vi "Get Attachments.vi"(6 "Authorization":T2[](array[typedef]), 8 "error in (no error)":errorcluster, 10 "Task GID":string) -> (0 "error out":errorcluster, 1 "data":T1(array[cluster]))   [LabVIEW 2016]
uses:
  <vilib>/addons/_JKI.lib/REST Client/classes/REST Client/HTTP Header.ctl
  <vilib>/addons/_JKI.lib/REST Client/classes/REST Client/REST Client.lvclass
  <vilib>/addons/_JKI.lib/Serialization/JSON/JKI JSON Serialization.lvlib
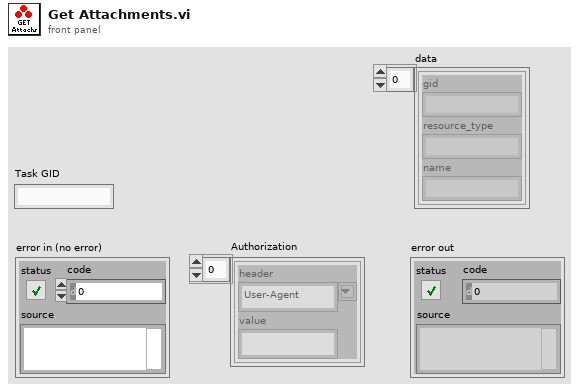
[diagram p1: front panel]
types:
  T1 = cluster{"gid":string, "resource_type":string, "name":string}[]
  T2 = typedef "REST Client.lvlib/REST Client.lvclass/HTTP Header.ctl" = cluster{"header":string, "value":string}
  T3 = cluster{"data":cluster{"gid":string, "resource_type":string, "name":string}[]}
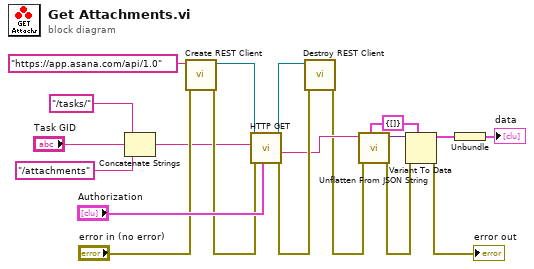
[diagram p0: block diagram]
diagram:
  w3 = T3 {"data"=[]}
  n1 = Concatenate Strings("/tasks/", "Task GID", "/attachments") -> (w14:string)
  n2 = call <vilib>:"Create REST Client.vi"("error in (no error)"="error in (no error)", "Base URL"="https://app.asana.com/api/1.0") -> ("error out"=w15:errorcluster, "REST Client out"=w17:refnum<class "REST Client.lvclass">)  [unwired: 8 in]
  n3 = call-dynamic "HTTP GET.vi"("request specific headers"="Authorization", "error in (no error)"=w15, "Path"=w14, "REST Client in"=w17) -> ("error out"=w10:errorcluster, "Response body"=w8:string, "REST Client out"=w9:refnum<class "REST Client.lvclass">)  [unwired: 2 in, 3 out]
  n4 = call-dynamic "Destroy REST Client.vi"("error in (no error)"=w10, "REST Client in"=w9) -> ("error out"=w7:errorcluster)  [unwired: 9 in]
  n5 = call <vilib>:"Unflatten From JSON String.vi"("Type and Defaults"=w3, "error in (no error)"=w7, "JSON String"=w8) -> ("error out"=w6:errorcluster, "Variant"=w4:variant)  [unwired: 7 in]
  n6 = Variant To Data(error in=w6, type=w3, Variant=w4) -> (data=w2:T3, error out=→"error out":errorcluster)
  n7 = Unbundle(w2) -> ("data"=→"data":T1)
